vi "Scale Image.vi"(8 "error in (no error)":errorcluster, 10 "Scale":cluster{"scale factor":dbl, "Scale":bool}, 11 "Refnum in":T1) -> (0 "error out":errorcluster, 3 "Refnum out":T1)   [LabVIEW 2013]
uses:
  <vilib>/vision/Image Controls.llb/IMAQ Image.ctl
  <vilib>/vision/NI_Vision_Development_Module.lvlib
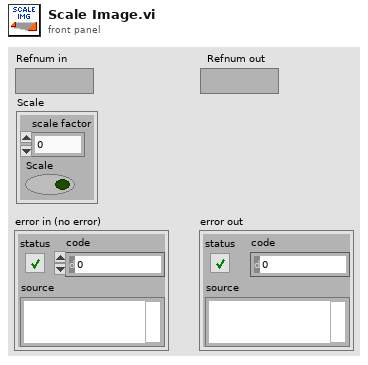
[diagram p1: front panel]
types:
  T1 = typedef "IMAQ Image.ctl" = refnum<image>
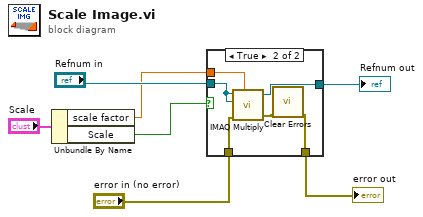
[diagram p0: block diagram]
diagram:
  n1 = Unbundle By Name("Scale") -> ("scale factor"=w2:dbl, "Scale"=w1:bool)
  n2 = case shown="True" w1 {
    tunnel: "Refnum in" -> [w9 w13]
    tunnel: w2 -> [_ w15]
    tunnel: [w9 w12] -> w6
    tunnel: "error in (no error)" -> [w8 w11]
    tunnel: [w8 w10] -> w5
    frame False {
    }
    frame True {
      n3 = call "IMAQ Multiply"("Image Src A"=w13, "Constant"=w15, "Image Dst"=w13, "error in (no error)"=w11) -> ("Image Dst Out"=w12:T1, "error out"=w14:errorcluster)  [unwired: 3 in]
      n4 = call <vilib>:"Clear Errors.vi"("error in (no error)"=w14) -> ("error out"=w10:errorcluster)  [unwired: 6 in]
    }
  }
  "Refnum out" <- w6
  "error out" <- w5
